vi "ArrayToProtocol.vi"(10 "Simulated Data":u16[](array[numeric]), 11 "Queue":refnum<queue>) -> ()   [LabVIEW 2013]
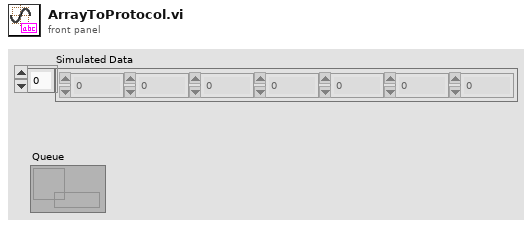
[diagram p1: front panel]
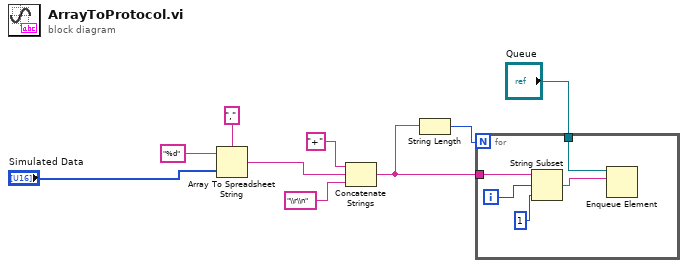
[diagram p0: block diagram]
diagram:
  n1 = Array To Spreadsheet String(delimiter (Tab)=",", array="Simulated Data", 3:"%d" ("format string")) -> (spreadsheet string=w5:string)
  n2 = Concatenate Strings("+" ("string"), w5, "\\r\\n" ("string")) -> (w2:string)
  n3 = String Length(string=w2) -> (length=w3:i32)
  n4 = for {
    N: w3 -> [_]
    tunnel: w2 -> [w14]
    tunnel: "Queue" -> [w12]
    i -> [w13]
    n5 = String Subset(string=w14, offset (0)=w13, length (rest)=1 ("length (rest)")) -> (substring=w11:string)
    n6 = Enqueue Element(queue=w12, element=w11) -> ()  [unwired: 2 in, 3 out]
  }
